vi "Choreo_TrajectoryState_New.vi"(5 "timestamp":dbl, 6 "angularVelocity":dbl, 7 "x":dbl, 8 "velocityY":dbl, 9 "velocityX":dbl, 10 "heading":dbl, 11 "y":dbl) -> (3 "ChoreoTrajectoryState":T1)   [LabVIEW 2019, in "ChoreoLib.lvlib"]
uses:
  ChoreoLib.lvlib
  TypeDef/ChoreoTrajectoryState.ctl
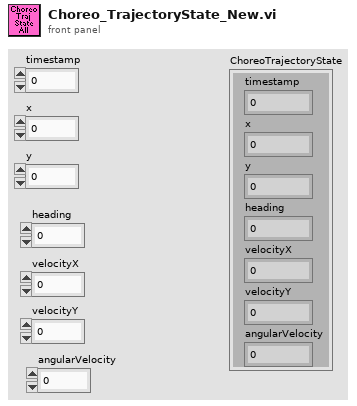
[diagram p1: front panel]
types:
  T1 = typedef "ChoreoLib.lvlib/ChoreoTrajectoryState.ctl" = cluster{"timestamp":dbl, "x":dbl, "y":dbl, "heading":dbl, "velocityX":dbl, "velocityY":dbl, "angularVelocity":dbl}
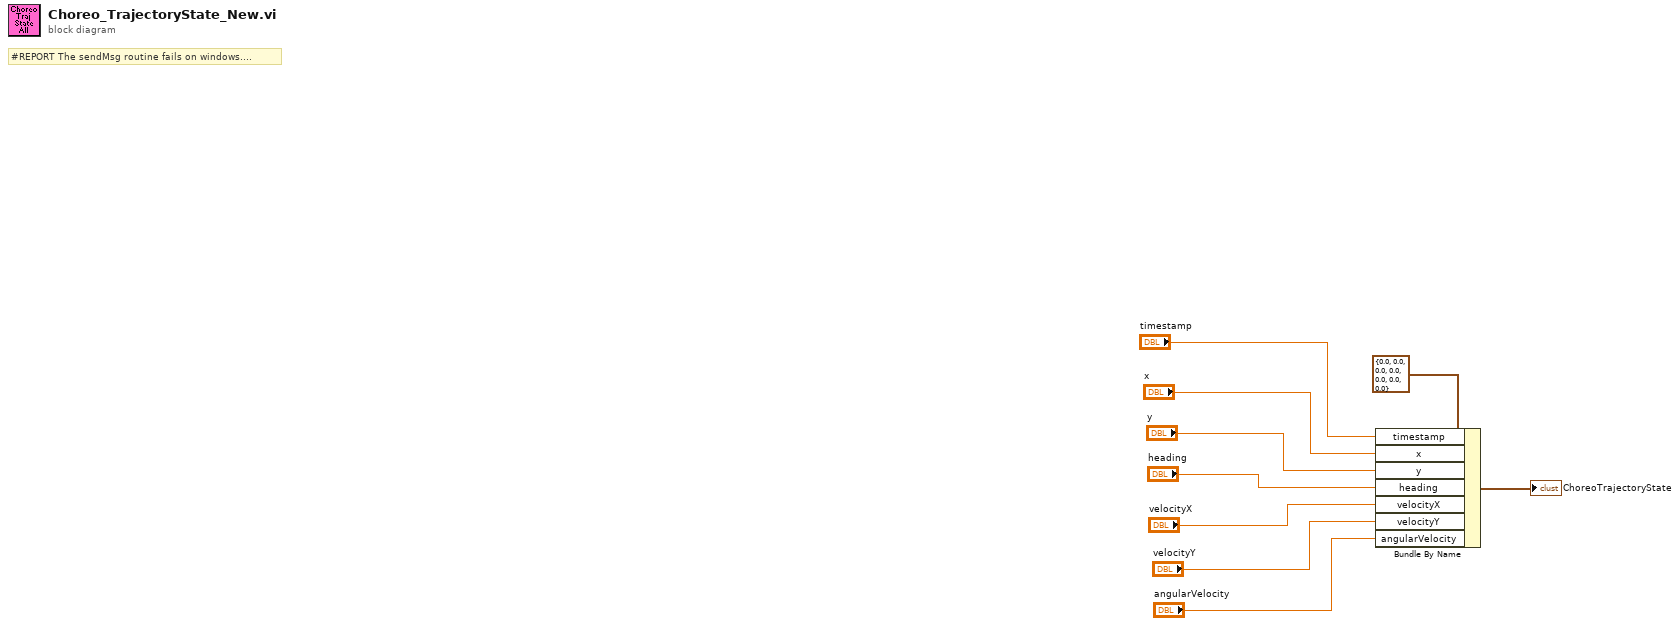
[diagram p0: block diagram]
diagram:
  # "#REPORT The sendMsg routine fails on windows...."
  n1 = Bundle By Name(cluster=T1 {"timestamp"=0.0, "x"=0.0, "y"=0.0, "heading"=0.0, "velocityX"=0.0, "velocityY"=0.0, "angularVelocity"=0.0} ("ChoreoTrajectoryState"), "timestamp"="timestamp", "x"="x", "y"="y", "heading"="heading", "velocityX"="velocityX", "velocityY"="velocityY", "angularVelocity"="angularVelocity") -> (→"ChoreoTrajectoryState":T1)
